vi "Low Level Find All.vi"(8 "error in (no error)":errorcluster) -> (0 "error out":errorcluster, 1 "specific error cleared?":bool, 2 "Array 2":string[](array[string]), 3 "Array":errorcluster[](array[cluster]), 4 "find list":string[](array[string]), 6 "List of Instruments":T1(array[cluster]))   [LabVIEW 2014, in "SetUp VIs.lvlib"]
uses:
  SetUp VIs.lvlib
  <vilib>/Instr/_visa.llb/VISA Find Search Mode.ctl
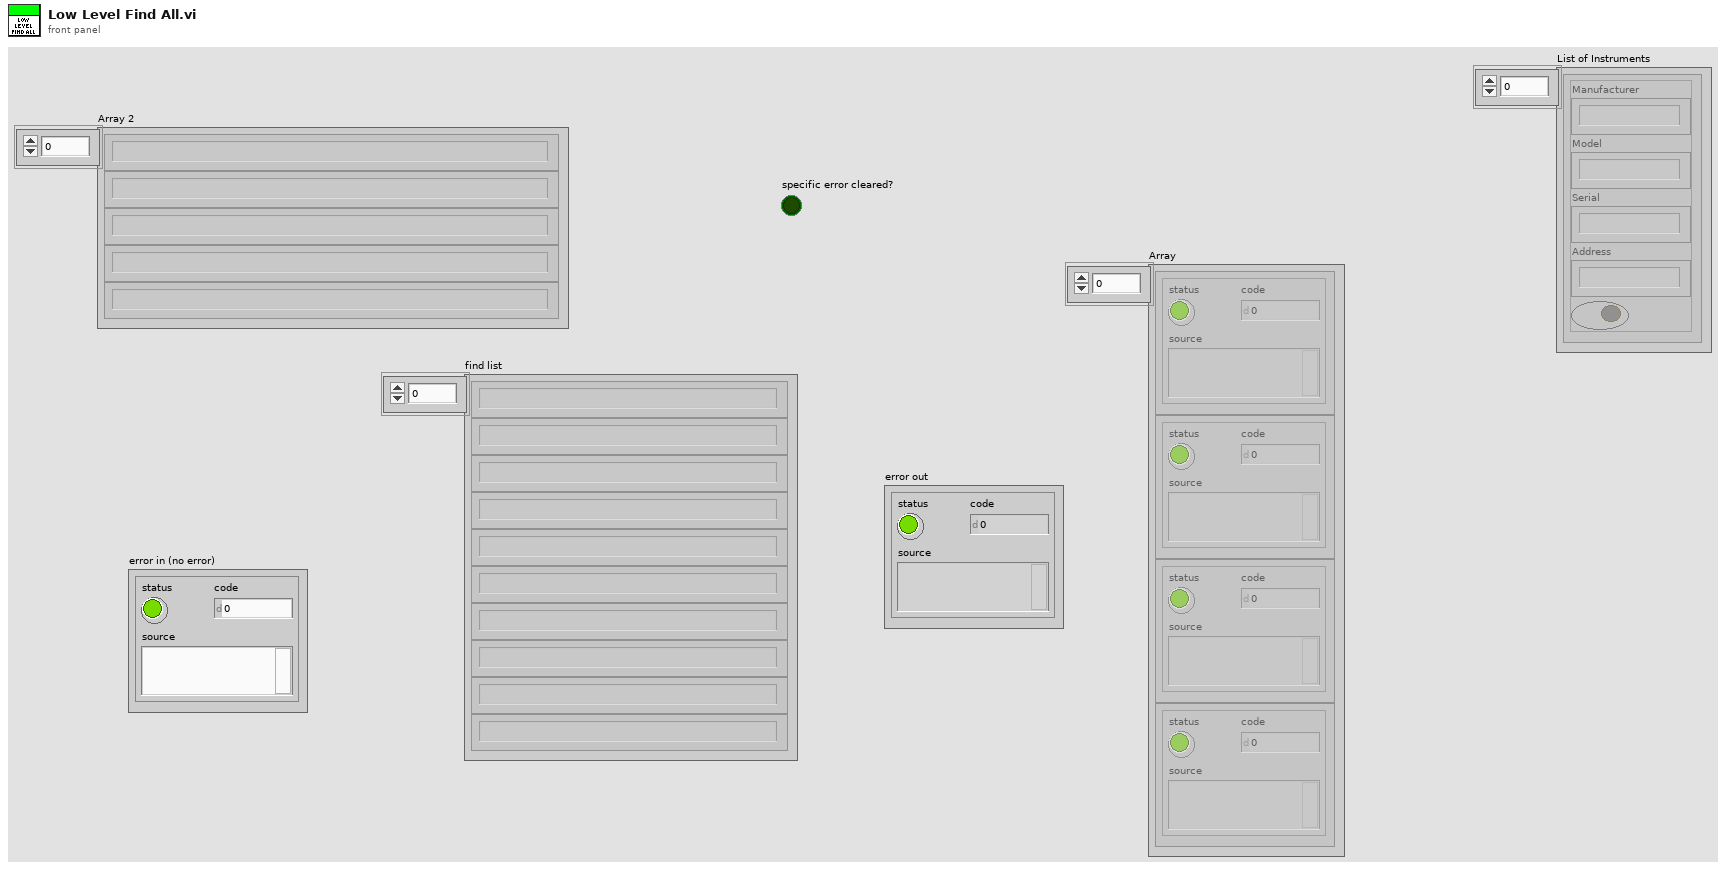
[diagram p1: front panel]
types:
  T1 = cluster{"Manufacturer":string, "Model":string, "Serial":string, "Address":string, "Boolean":bool}[]
  T2 = typedef "VISA Find Search Mode.ctl" = u32
  T3 = cluster{"Manufacturer":string, "Model":string, "Serial":string, "Address":string, bool}[]
  T4 = cluster{"Manufacturer":string, "Model":string, "Serial":string, "Address":string, bool}
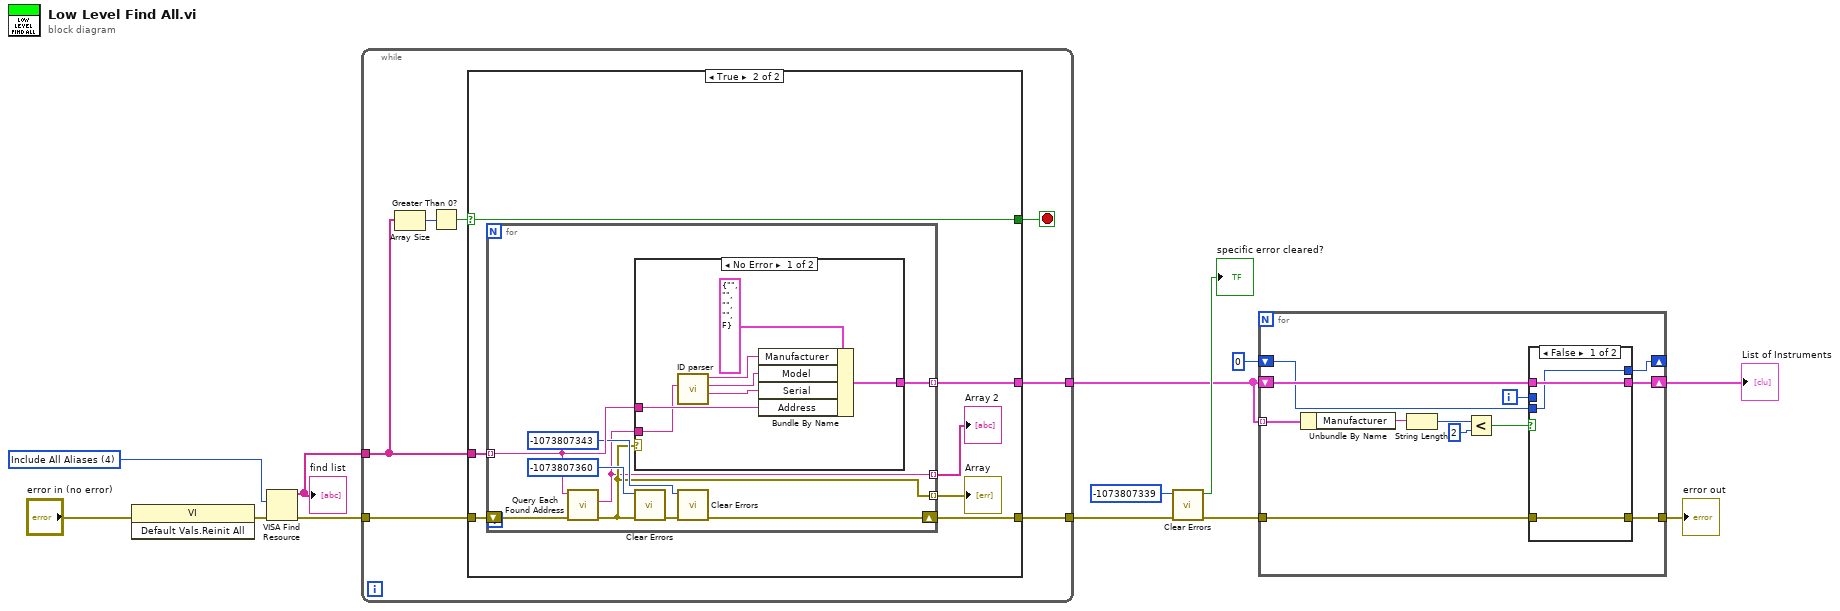
[diagram p0: block diagram]
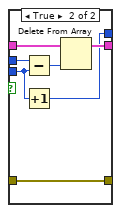
[diagram p2: hidden frame]
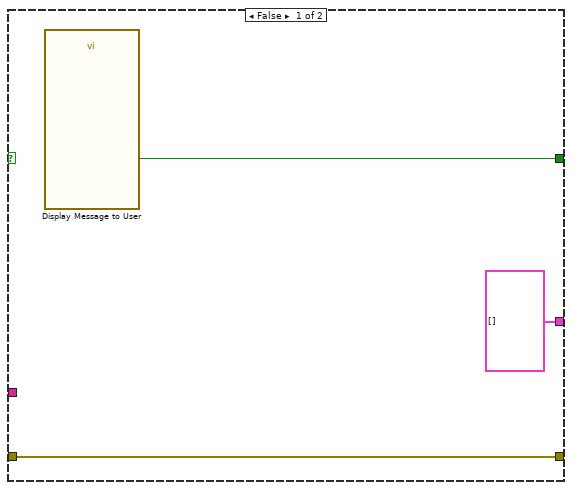
[diagram p3: hidden frame]
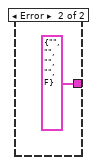
[diagram p4: hidden frame]
diagram:
  w4 = T2 4 items=["Canonical Names Only"=0, "Aliases Only"=2, "Include Matching Aliases"=3, "Include All Aliases"=4] ("Search Mode")
  n1 = invoke class="VI" method="Default Vals.Reinit All"(error in="error in (no error)") -> (error out=w1:errorcluster)  [unwired: 2 in, 2 out]
  n2 = VISA Find Resource(8:w1, 10:w4) -> (0:w2:errorcluster, 3:w5:string[])  [unwired: 1 in, 1 out]
  "find list" <- w5
  n3 = while {
    tunnel: w5 -> [w17]
    tunnel: [w20] -> w10
    tunnel: [w18] -> w6
    tunnel: w2 -> [w19]
    stop <- w14 stop-if-true
    n4 = Array Size(array=w17) -> (size(s)=w16:i32)
    n5 = Greater Than 0?(x=w16) -> (x > 0?=w15:bool)
    n6 = case shown="True" w15 {
      selector: w15 -> [_ w26]
      tunnel: w17 -> [_ w30]
      tunnel: [w22 w29] -> w20
      tunnel: w19 -> [w22 w28]
      tunnel: [T3 [] w27] -> w18
      tunnel: [w23 w26] -> w14
      frame False {
        n7 = call "Display Message to User"() -> ("OK"=w23:bool)  [unwired: 10 in, 1 out]
      }
      frame True {
        n8 = for {
          tunnel: w30 -> [w39] mode=indexing
          tunnel: [w38] -> w27 mode=indexing
          shift-right: [w33] -> w29
          shift-left: w28 -> [w37]
          tunnel: [w32] -> w25 mode=indexing
          tunnel: [w31] -> w24 mode=indexing
          n9 = call "Query Each Found Address.vi"("error in (no error) 2"=w37, "Address"=w39) -> ("error out (no error)"=w32:errorcluster, "read buffer"=w31:string)  [unwired: 8 in]
          n10 = case shown="No Error" w32 {
            tunnel: w39 -> [w46 _]
            tunnel: [w45 T4 {"Manufacturer"="", "Model"="", "Serial"="", "Address"="", FALSE} ("Instrument")] -> w38
            tunnel: w31 -> [w40 _]
            frame No Error {
              n11 = call "ID parser.vi"("Input String"=w40) -> ("Serial"=w42:string, "Model"=w43:string, "Manufacturer"=w44:string)  [unwired: 8 in]
              n12 = Bundle By Name(cluster=T4 {"Manufacturer"="", "Model"="", "Serial"="", "Address"="", FALSE} ("Instrument"), "Manufacturer"=w44, "Model"=w43, "Serial"=w42, "Address"=w46) -> (w45:T4)
            }
            frame Error {
            }
          }
          n13 = call <vilib>:"Clear Errors.vi"("error in (no error)"=w32, "specific error code to clear (0: all)"=-1073807360) -> ("error out"=w35:errorcluster)  [unwired: 4 in, 1 out]
          n14 = call <vilib>:"Clear Errors.vi"("error in (no error)"=w35, "specific error code to clear (0: all)"=-1073807343) -> ("error out"=w33:errorcluster)  [unwired: 4 in, 1 out]
        }
        "Array" <- w25
        "Array 2" <- w24
      }
    }
  }
  n15 = call <vilib>:"Clear Errors.vi"("error in (no error)"=w10, "specific error code to clear (0: all)"=-1073807339) -> ("error out"=w11:errorcluster, "specific error cleared?"=→"specific error cleared?":bool)  [unwired: 4 in]
  n16 = for {
    tunnel: w6 -> [w59] mode=indexing
    shift-right: [w55] -> w8
    shift-left: w6 -> [w57]
    tunnel: w11 -> [w54]
    tunnel: [w53] -> w7
    shift-right: [w48] -> _
    shift-left: 0 -> [w49]
    i -> [w56]
    n17 = Unbundle By Name(w59) -> ("Manufacturer"=w58:string)
    n18 = String Length(string=w58) -> (length=w50:i32)
    n19 = Less?(x=w50, y=2) -> (x < y?=w52:bool)
    n20 = case shown="False" w52 {
      tunnel: w57 -> [w61 w69]
      tunnel: w56 -> [_ w66]
      tunnel: [w61 w68] -> w55
      tunnel: w54 -> [w62 w67]
      tunnel: [w62 w67] -> w53
      tunnel: w49 -> [w60 w64]
      tunnel: [w60 w63] -> w48
      frame False {
      }
      frame True {
        n21 = Subtract(x=w66, y=w64) -> (x-y=w65:i32)
        n22 = Increment(x=w64) -> (x+1=w63:i32)
        n23 = Delete From Array(array=w69, index=w65) -> (array with subset deleted=w68:T3)  [unwired: 1 in, 1 out]
      }
    }
  }
  "List of Instruments" <- w8
  "error out" <- w7
